vi "SubVI Modulation.vi"(8 "载波信号采样信息":cluster{"Fs":dbl, "#s":dbl}={"Fs"=1000.0, "#s"=1000.0} caption="采样信息" {"Fs" format="%.2p"}, 9 "载波频率(Hz)":dbl(slide) scale=0.0..1000000.0 scale format="%#_4p", 10 "FM 频偏(Hz)":dbl(slide) scale=0.0..200000.0 scale format="%#_4p", 11 "基带信号":waveform(dbl)) -> (1 "FFT (功率谱)":dynamicdata(graph)=[{"t0"=timestamp(0 s since 1904-01-01), "dt"=1e-07, "Y"=array[2000 elements]}, {"t0"=timestamp(0 s since 1904-01-01), "dt"=1e-07, "Y"=array[2000 elements]}], 2 "频率调制波":waveform(dbl)(graph), 3 "载波信号":waveform(dbl)(graph))   [LabVIEW 2015]
uses:
  <vilib>/express/express analysis/Spectral/Block/exnSpectralBlock spectral measurements power poly.vi
  <vilib>/express/express analysis/Spectral/Block/exnSpectralBlock spectral measurements power DDT.vi
  <vilib>/express/express analysis/Spectral/XNode/ExpressSpectralMeasurementsBlockNode.xnode
  <vilib>/measure/NI_MABase.lvlib
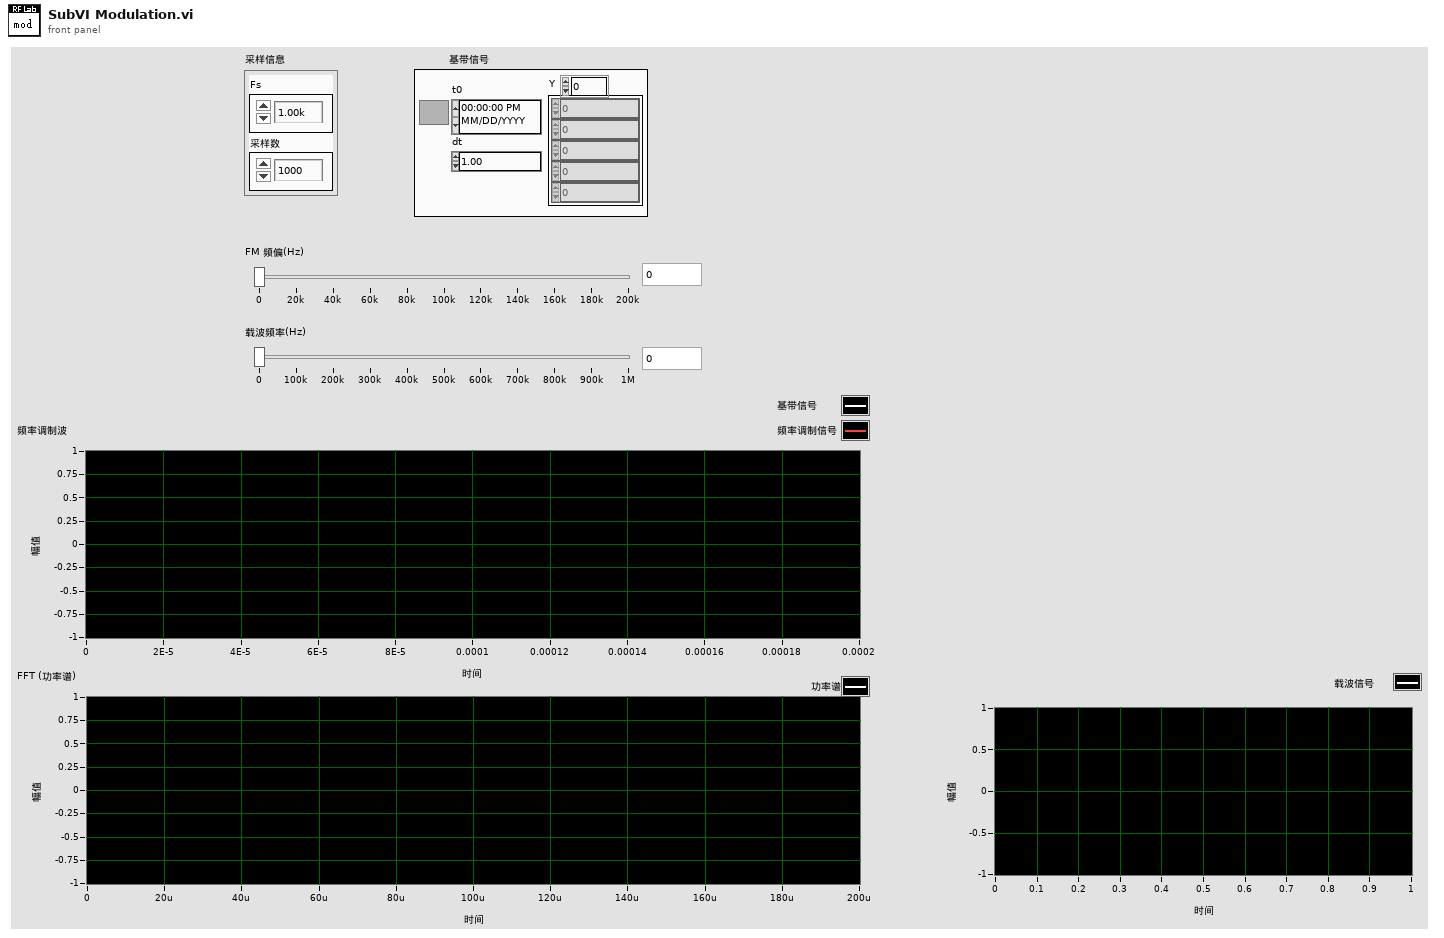
[diagram p1: front panel]
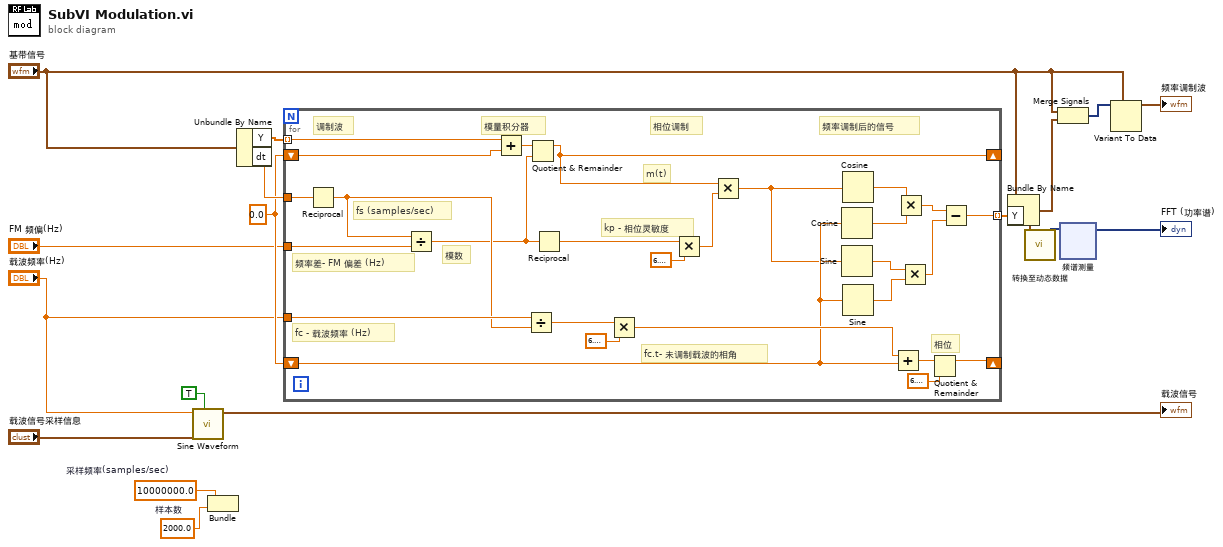
[diagram p0: block diagram]
diagram:
  w10 = 0.0
  w11 = 10000000.0  # 采样频率(samples/sec)
  w12 = 2000.0  # 样本数
  n1 = call <vilib>:"Sine Waveform.vi"("sampling info"="载波信号采样信息", "reset signal"=TRUE, "frequency"="载波频率(Hz)") -> ("signal out"=→"载波信号":waveform(dbl))  [unwired: 7 in, 1 out]
  n2 = Bundle("采样频率(samples/sec)"=w11, "样本数"=w12) -> ()  [unwired: 1 in, 1 out]
  n3 = Unbundle By Name("基带信号") -> ("Y"=w17:dbl[], "dt"=w14:dbl)
  n4 = for {
    tunnel: w14 -> [w44]
    tunnel: "FM 频偏(Hz)" -> [w43]
    shift-right: [w28] -> _
    shift-left: w10 -> [w27]
    tunnel: w17 -> [w26] mode=indexing
    tunnel: "载波频率(Hz)" -> [w40]
    tunnel: [w35] -> w15 mode=indexing
    shift-right: [w31] -> _
    shift-left: w10 -> [w24]
    # "fc.t- 未调制载波的相角"
    # "m(t)"
    # "调制波"
    # "fc - 载波频率 (Hz)"
    # "频率差- FM 偏差 (Hz)"
    # "相位"
    # "频率调制后的信号"
    # "相位调制"
    # "kp - 相位灵敏度"
    # "模量积分器"
    # "模数"
    # "fs (samples/sec)"
    n5 = Reciprocal(x=w44) -> (1/x=w39:dbl)
    n6 = Divide(x=w39, y=w43) -> (x/y=w29:dbl)
    n7 = Add(x=w26, y=w27) -> (x+y=w30:dbl)
    n8 = Divide(x=w40, y=w39) -> (x/y=w37:dbl)
    n9 = Quotient & Remainder(x=w30, y=w29) -> (x-y*floor(x/y)=w28:dbl)  [unwired: 1 out]
    n10 = Reciprocal(x=w29) -> (1/x=w18:dbl)
    n11 = Multiply(x=w37, y=6.283185307179586) -> (x*y=w34:dbl)
    n12 = Multiply(x=w18, y=6.283185307179586) -> (x*y=w41:dbl)
    n13 = Multiply(x=w28, y=w41) -> (x*y=w19:dbl)
    n14 = Cosine(x=w24) -> (cos(x)=w21:dbl)
    n15 = Sine(x=w19) -> (sin(x)=w20:dbl)
    n16 = Cosine(x=w19) -> (cos(x)=w22:dbl)
    n17 = Sine(x=w24) -> (sin(x)=w23:dbl)
    n18 = Add(x=w34, y=w24) -> (x+y=w33:dbl)
    n19 = Multiply(x=w22, y=w21) -> (x*y=w36:dbl)
    n20 = Multiply(x=w20, y=w23) -> (x*y=w25:dbl)
    n21 = Quotient & Remainder(x=w33, y=6.283185307179586) -> (x-y*floor(x/y)=w31:dbl)  [unwired: 1 out]
    n22 = Subtract(x=w36, y=w25) -> (x-y=w35:dbl)
  }
  n23 = Bundle By Name(cluster="基带信号", "Y"=w15) -> (w8:waveform(dbl))
  n24 = call "转换至动态数据"("Waveform"=w8) -> ("Dynamic Data Type"=w6:dynamicdata)  [unwired: 3 in]
  n25 = Merge Signals("基带信号", w8) -> (w16:dynamicdata)
  n26 = xnode "频谱测量"("信号"=w6) -> ("Power Spectrum"=→"FFT (功率谱)":dynamicdata)  [unwired: 1 in, 1 out]
  n27 = Variant To Data(type="基带信号", Variant=w16) -> (data=→"频率调制波":waveform(dbl))  [unwired: 1 in, 1 out]
